vi "DriveNetwork.vi"   [LabVIEW 2020]
uses:
  DriveGlobals.vi
  <vilib>/Rock Robotics/Network Tables/NT Write Number.vi
  <vilib>/Rock Robotics/Network Tables/NT Write Boolean.vi
  <vilib>/Rock Robotics/Network Tables/NT Read Number.vi
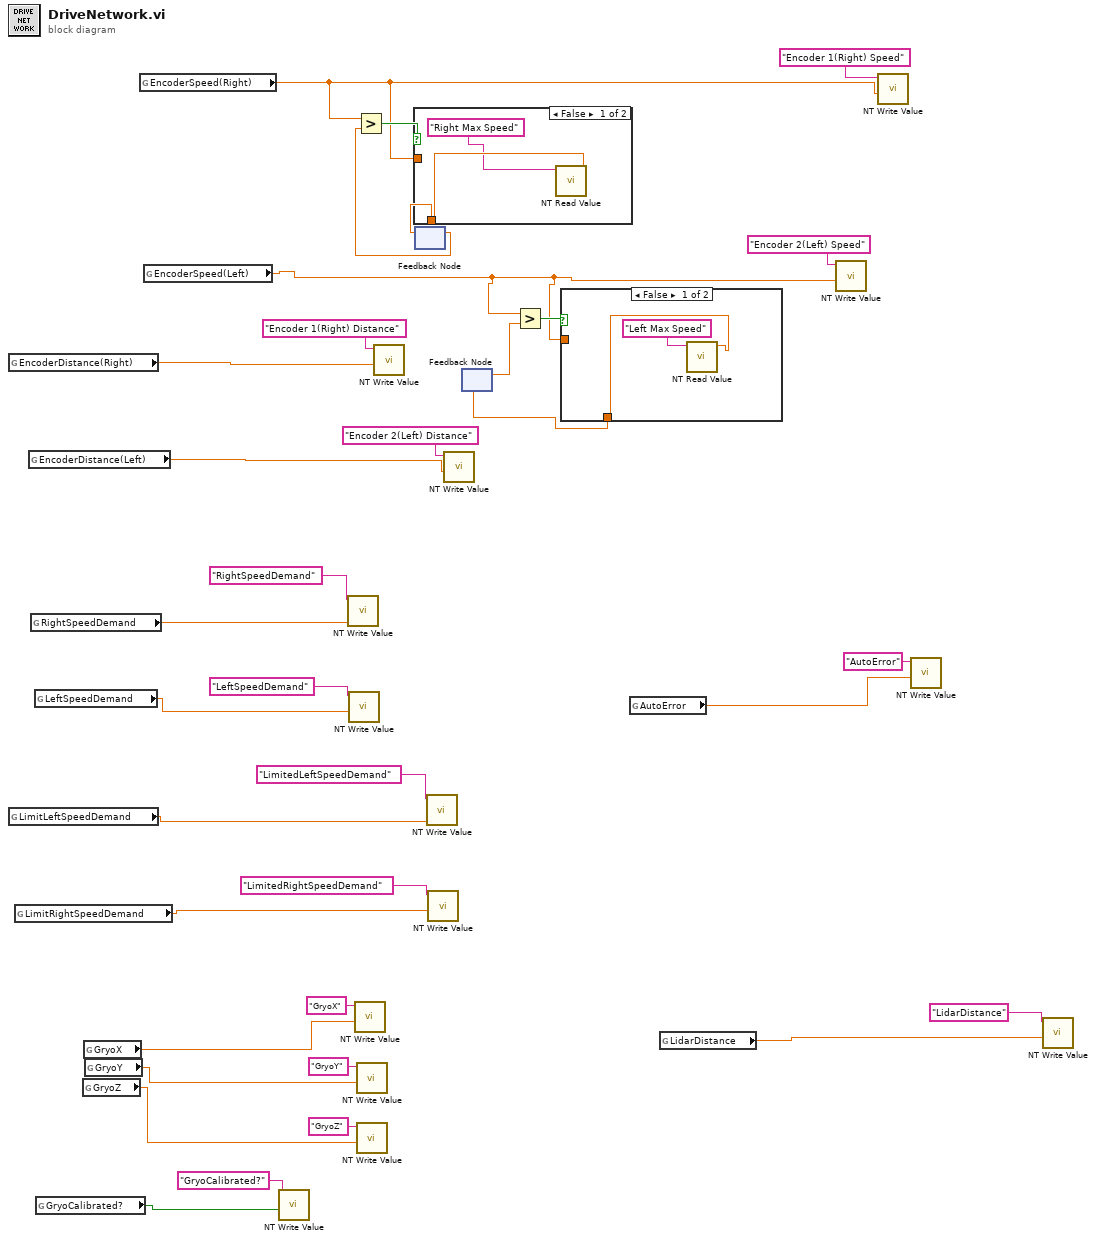
[diagram p0: block diagram]
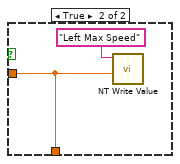
[diagram p2: hidden frame]
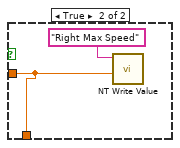
[diagram p3: hidden frame]
diagram:
  n1 = global read "DriveGlobals.vi" "EncoderDistance(Right)"() -> (w15:dbl)
  n2 = global read "DriveGlobals.vi" "LimitLeftSpeedDemand"() -> (w23:dbl)
  n3 = global read "DriveGlobals.vi" "LimitRightSpeedDemand"() -> (w24:dbl)
  n4 = global read "DriveGlobals.vi" "EncoderDistance(Left)"() -> (w16:dbl)
  n5 = global read "DriveGlobals.vi" "RightSpeedDemand"() -> (w30:dbl)
  n6 = global read "DriveGlobals.vi" "LeftSpeedDemand"() -> (w29:dbl)
  n7 = global read "DriveGlobals.vi" "GryoCalibrated?"() -> (w6:bool)
  n8 = global read "DriveGlobals.vi" "GryoZ"() -> (w7:dbl)
  n9 = global read "DriveGlobals.vi" "GryoX"() -> (w9:dbl)
  n10 = global read "DriveGlobals.vi" "GryoY"() -> (w8:dbl)
  n11 = global read "DriveGlobals.vi" "EncoderSpeed(Right)"() -> (w14:dbl)
  n12 = global read "DriveGlobals.vi" "EncoderSpeed(Left)"() -> (w13:dbl)
  n13 = call-poly <vilib>:"NT Write Value.vi"("Boolean"=w6, "Name"="GryoCalibrated?") -> ()  [unwired: 9 in, 1 out]
  n14 = call-poly <vilib>:"NT Write Value.vi"("Numeric"=w30, "Name"="RightSpeedDemand") -> ()  [unwired: 9 in, 1 out]
  n15 = call-poly <vilib>:"NT Write Value.vi"("Numeric"=w29, "Name"="LeftSpeedDemand") -> ()  [unwired: 9 in, 1 out]
  n16 = call-poly <vilib>:"NT Write Value.vi"("Numeric"=w9, "Name"="GryoX") -> ()  [unwired: 9 in, 1 out]
  n17 = call-poly <vilib>:"NT Write Value.vi"("Numeric"=w8, "Name"="GryoY") -> ()  [unwired: 9 in, 1 out]
  n18 = call-poly <vilib>:"NT Write Value.vi"("Numeric"=w7, "Name"="GryoZ") -> ()  [unwired: 9 in, 1 out]
  n19 = call-poly <vilib>:"NT Write Value.vi"("Numeric"=w15, "Name"="Encoder 1(Right) Distance") -> ()  [unwired: 9 in, 1 out]
  n20 = feedback #1() -> (w19:dbl)  [unwired: 1 in]
  n21 = Greater?(x=w14, y=w19) -> (0:w22:bool)
  n22 = case shown="False" w22 {
    tunnel: w14 -> [_ w37]
    tunnel: [w36 w37] -> w20
    frame False {
      n23 = call-poly <vilib>:"NT Read Value.vi"("Name"="Right Max Speed") -> ("Numeric"=w36:dbl)  [unwired: 9 in, 1 out]
    }
    frame True {
      n24 = call-poly <vilib>:"NT Write Value.vi"("Numeric"=w37, "Name"="Right Max Speed") -> ()  [unwired: 9 in, 1 out]
    }
  }
  n25 = feedback-in #1(w20) -> ()
  n26 = call-poly <vilib>:"NT Write Value.vi"("Numeric"=w23, "Name"="LimitedLeftSpeedDemand") -> ()  [unwired: 9 in, 1 out]
  n27 = call-poly <vilib>:"NT Write Value.vi"("Numeric"=w24, "Name"="LimitedRightSpeedDemand") -> ()  [unwired: 9 in, 1 out]
  n28 = call-poly <vilib>:"NT Write Value.vi"("Numeric"=w16, "Name"="Encoder 2(Left) Distance") -> ()  [unwired: 9 in, 1 out]
  n29 = feedback #2() -> (w17:dbl)  [unwired: 1 in]
  n30 = Greater?(x=w13, y=w17) -> (0:w21:bool)
  n31 = case shown="False" w21 {
    tunnel: w13 -> [_ w41]
    tunnel: [w40 w41] -> w18
    frame False {
      n32 = call-poly <vilib>:"NT Read Value.vi"("Name"="Left Max Speed") -> ("Numeric"=w40:dbl)  [unwired: 9 in, 1 out]
    }
    frame True {
      n33 = call-poly <vilib>:"NT Write Value.vi"("Numeric"=w41, "Name"="Left Max Speed") -> ()  [unwired: 9 in, 1 out]
    }
  }
  n34 = feedback-in #2(w18) -> ()
  n35 = global read "DriveGlobals.vi" "AutoError"() -> (w3:dbl)
  n36 = global read "DriveGlobals.vi" "LidarDistance"() -> (w1:dbl)
  n37 = call-poly <vilib>:"NT Write Value.vi"("Numeric"=w13, "Name"="Encoder 2(Left) Speed") -> ()  [unwired: 9 in, 1 out]
  n38 = call-poly <vilib>:"NT Write Value.vi"("Numeric"=w14, "Name"="Encoder 1(Right) Speed") -> ()  [unwired: 9 in, 1 out]
  n39 = call-poly <vilib>:"NT Write Value.vi"("Numeric"=w3, "Name"="AutoError") -> ()  [unwired: 9 in, 1 out]
  n40 = call-poly <vilib>:"NT Write Value.vi"("Numeric"=w1, "Name"="LidarDistance") -> ()  [unwired: 9 in, 1 out]
